vi "Test Apply Filter only Once.vi"(8 "error in (no error)":errorcluster, 11 "Test Case In":refnum<class "Debug Log Test.lvclass">) -> (0 "error out":errorcluster, 3 "Test Case Out":refnum<class "Debug Log Test.lvclass">)   [LabVIEW 2020, in "Debug Log Test.lvclass"]
uses:
  Debug Log Test.lvclass
  C:/Program Files (x86)/National Instruments/LabVIEW 2020/vi.lib/Astemes/LUnit/Test Case.lvclass
  source/Debug Log/Debug Log.lvclass
  <vilib>/Astemes/LUnit/Test Case.lvclass/Test Case.ctl
  <vilib>/Astemes/LUnit/LUnit Assertion Result.lvclass/LUnit Assertion Result.ctl
  <vilib>/Astemes/LUnit/LUnit Test Case Result.lvclass/LUnit Test Case Result.ctl
  <vilib>/Astemes/LUnit/LUnit Method Result.lvclass/LUnit Method Result.ctl
  01074fa8-ee8a-411d-bc8b-fc92c4f90959.vi
  <vilib>/Astemes/LUnit/Palette/Pass.vi
  <vilib>/Astemes/LUnit/Palette/Fail.vi
  <vilib>/Astemes/LUnit/Compare Variants.vi
  <vilib>/Astemes/LUnit/Describe Comparison.vi
  <vilib>/Astemes/LUnit/Set Assertion Type.vi
  <vilib>/Astemes/LUnit/Add test result.vi
  <vilib>/Astemes/LUnit/LUnit Write Passed.vi
  <vilib>/Astemes/LUnit/LUnit Write Message.vi
  <vilib>/Astemes/LUnit/LUnit Write Description.vi
  <vilib>/Astemes/LUnit/Variant to string.vi
  <vilib>/Astemes/LUnit/LUnit Write Assertion Type.vi
  <vilib>/Astemes/LUnit/LUnit Record Assertion Result.vi
  <vilib>/Astemes/LUnit/LUnit Aggregate Assertion Results.vi
  <vilib>/Astemes/LUnit/Assertion Result/LUnit Read Status.vi
  <vilib>/Astemes/LUnit/LUnit Read Message.vi
  <vilib>/Astemes/LUnit/LUnit Read Description.vi
  <vilib>/Astemes/LUnit/Method Result/LUnit Merge Status.vi
  <vilib>/Astemes/LUnit/LUnit Concatenate result strings.vi
  source/Mock Filter/Mock Filter.lvclass
  C:/Users/anton/Documents/GitHub/triarc-debugger/source/Filter/Filter.lvclass
  <vilib>/Utility/Data Type/Get Type Information.vi
  <vilib>/Utility/LVClass/Get LV Class Name.vi
  <vilib>/Astemes/LUnit/LUnit Assertion Result.lvclass
  Debug Log Test.lvclass/Debug Log Test.ctl
  source/Debug Data/Debug Data.lvclass
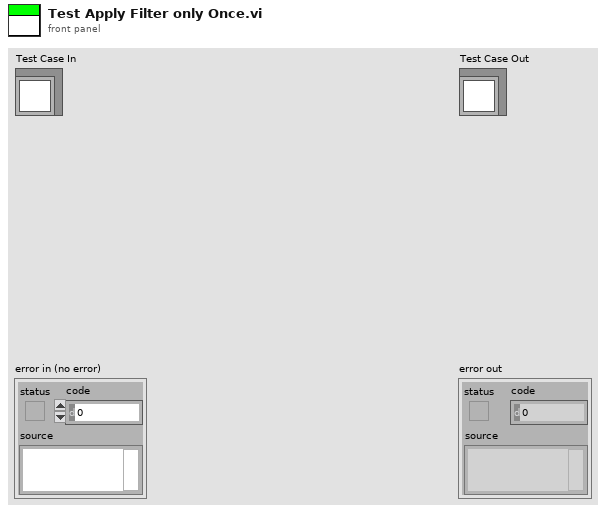
[diagram p1: front panel]
types:
  T1 = cluster{"Action":string, "Call Chain":string, "Process":string, "Message":string, "Message Data":variant, "Time":u32}[]
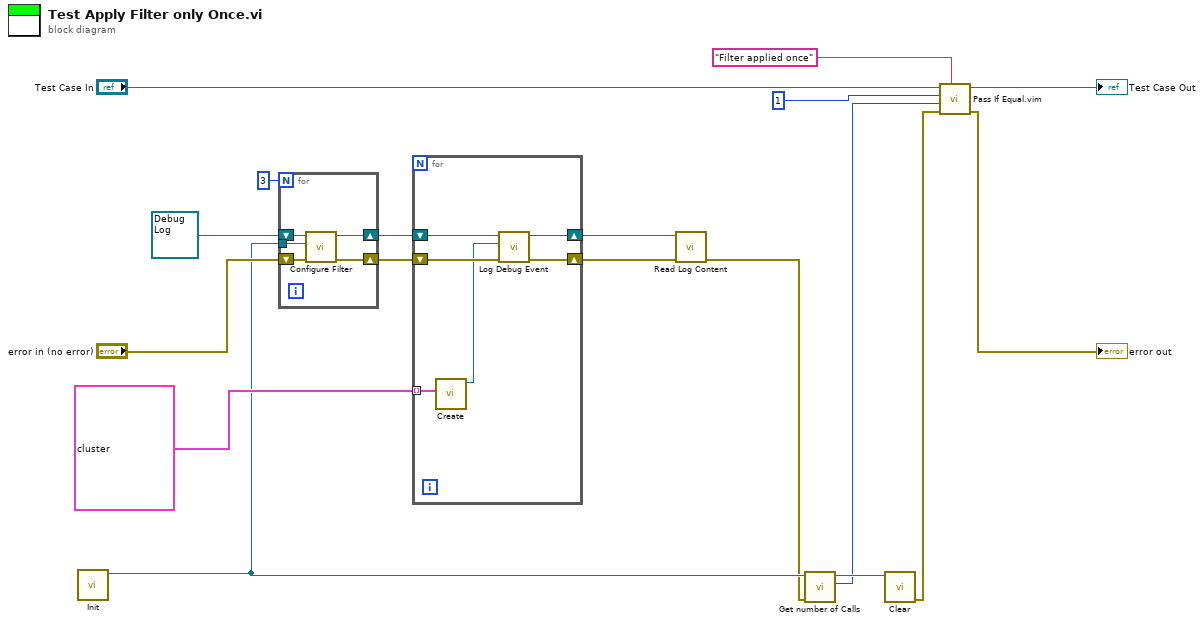
[diagram p0: block diagram]
diagram:
  n1 = call "Init.vi"() -> ("Mock Filter out"=w6:refnum<class "Mock Filter.lvclass">)  [unwired: 10 in, 1 out]
  n2 = for {
    N: 3 -> [_]
    tunnel: w6 -> [w19]
    shift-right: [w22] -> w9
    shift-left: "error in (no error)" -> [w23]
    shift-right: [w20] -> w7
    shift-left: refnum<class "Debug Log.lvclass"> refnum ("Debug Log.lvclass") -> [w21]
    n3 = call "Configure Filter.vi"("error in (no error)"=w23, "Filter"=w19, "Debug Log In"=w21) -> ("error out"=w22:errorcluster, "Debug Log Out"=w20:refnum<class "Debug Log.lvclass">)  [unwired: 7 in]
  }
  n4 = for {
    tunnel: T1 [{"Action"="", "Call Chain"="", "Process"="", "Message"="1", "Message Data"=variant, "Time"=0}, {"Action"="", "Call Chain"="", "Process"="", "Message"="2", "Message Data"=variant, "Time"=0}, {"Action"="", "Call Chain"="", "Process"="", "Message"="3", "Message Data"=variant, "Time"=0}] ("Debug Data Cluster") -> [w25] mode=indexing
    shift-right: [w28] -> w10
    shift-left: w7 -> [w29]
    shift-right: [w26] -> w16
    shift-left: w9 -> [w27]
    n5 = call "Create.vi"("Debug Data Cluster"=w25) -> ("Debug Data out"=w24:refnum<class "Debug Data.lvclass">)  [unwired: 9 in, 1 out]
    n6 = call "Log Debug Event.vi"("error in (no error)"=w27, "Debug Data.lvclass"=w24, "Debugger in"=w29) -> ("error out"=w26:errorcluster, "Debugger out"=w28:refnum<class "Debug Log.lvclass">)  [unwired: 7 in]
  }
  n7 = call "Read Log Content.vi"("error in (no error)"=w16, "Debug Log In"=w10) -> ("error out"=w3:errorcluster)  [unwired: 7 in, 2 out]
  n8 = call "Get number of Calls.vi"("error in (no error)"=w3, "Mock Filter in"=w6) -> ("Number of Calls"=w4:i32, "Mock Filter out"=w5:refnum<class "Mock Filter.lvclass">)  [unwired: 7 in, 1 out]
  n9 = call "Clear.vi"("Mock Filter in"=w5) -> ("error out"=w2:errorcluster)  [unwired: 9 in, 1 out]
  n10 = call "Pass If Equal.vim"("Description"="Filter applied once", "error in (no error)"=w2, "Actual"=w4, "Expected"=1 ("size(s)"), "LUnit Test Case In"="Test Case In") -> ("error out"=→"error out":errorcluster, "LUnit Test Case Out"=→"Test Case Out":refnum<class "Debug Log Test.lvclass">)  [unwired: 5 in]
